vi "Test email.vi"() -> ()   [LabVIEW 2016]
uses:
  <vilib>/smtpClient/LabVIEWSMTPClient.lvlib
  <vilib>/smtpClient/Set Message Text Html.vi
panel:
  in  "use TLS (false)":bool
  in  "error in (no error)":errorcluster
  in  "password":string
  in  "username":string
  in  "from":string
  in  "server address":string
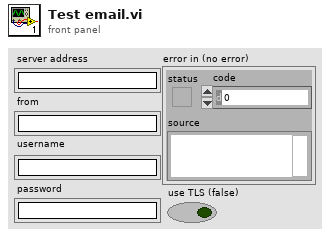
[diagram p1: front panel]
types:
  T1 = typedef "LabVIEWSMTPClient.lvlib/SmtpClientHandle.ctl" = refnum<k1>
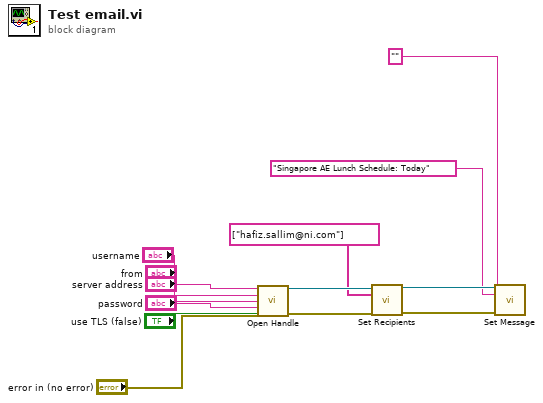
[diagram p0: block diagram]
diagram:
  n1 = call <vilib>:"Open Handle.vi"("server address"="server address", "from"="from", "username"="username", "password"="password", "error in (no error)"="error in (no error)", "use TLS (false)"="use TLS (false)") -> ("handle out"=w7:T1, "error out"=w6:errorcluster)  [unwired: 8 in]
  n2 = call <vilib>:"Set Recipients.vi"("handle in"=w7, "to"=string[] ["hafiz.sallim@ni.com"], "error in (no error)"=w6) -> ("handle out"=w4:T1, "error out"=w3:errorcluster)  [unwired: 11 in]
  n3 = call-poly <vilib>:"Set Message.vi"("handle in"=w4, "subject"="Singapore AE Lunch Schedule: Today", "html message"="", "error in (no error)"=w3) -> ()  [unwired: 10 in, 2 out]
